vi "適應性控制_連續取樣版(實際控制).vi"() -> ()   [LabVIEW 2010]
panel:
  out "A1_input_x(t)":dbl(graph)
  in  "milliseconds to wait":u32
  out "Numeric":dbl
  out "while平均運行時間(ms)":dbl
  in  "number of samples(不可低於2)":i32=100 min=2
  in  "rate":dbl=1000.0
  out "收斂時間(s)":dbl
  out "收斂燈":bool
  in  "ERR誤差低於多少V亮燈":dbl=0.05
  out "ERR message":string=" INSTRUCTIONS:\r\rNormal Use:  When using subVIs that incorporate the error in/error out (or error I/O) structure, place this handler where you want to inform the user of an error, typically at the end of the I/O data path, as the last action of the program.  If the error in error? is ERROR, the handler creates a message describing the error and its source.  If the type of dialog = 1 (default), the message is displayed to the user, who can only acknowedge it.  If the type = 2, the user can acknowledge the message or abort execution; aborting a program with active I/O is not recommended.  If the type = 0, no message is displayed; this is used to process the error programmatically, and the error out cluster elements are wired to individual terminals for that reason.  \r\rOther Use:\n\r\nlocal testing.  To test the error code of a subVI or function that does not have the error I/O structure, you can wire its error code and a source string to the local error code and error source inputs.  If error in error? indicates no error and error code is not equal to 0, the local code and source are substituted for the error in values, and error? is set TRUE (ERROR)."
  out "理想系統與FIR輸出":cluster{dbl, dbl}(graph)
  out "system輸出":dbl
  out "A0_input_x(t)":dbl(graph)
  out "ERR":dbl(graph)
  out "權重函數向量":dbl[](array[numeric])
  in  "order":i32=8
  out "LMS":dbl[](graph)
  out "FIR輸出":dbl
  in  "Stop Button":bool
  in  "u(收斂係數)":dbl=0.005
  # "A0:模擬輸入 pulse_output 1"
  # "A1:理想系統 pulse_output 2"
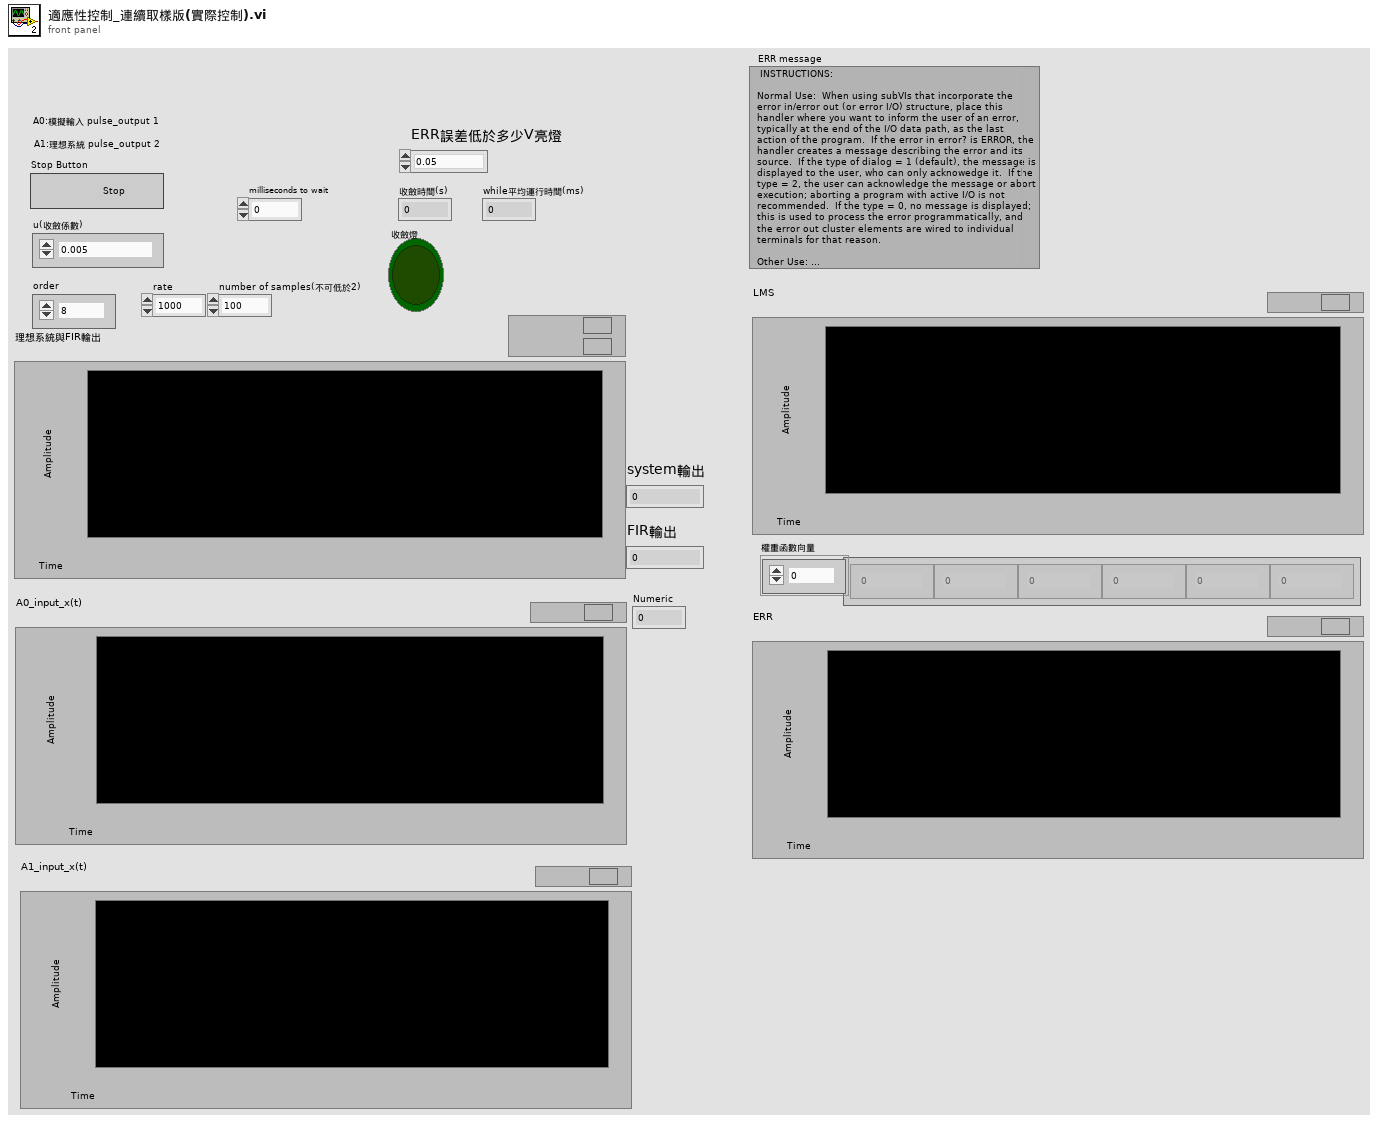
[diagram p1: front panel]
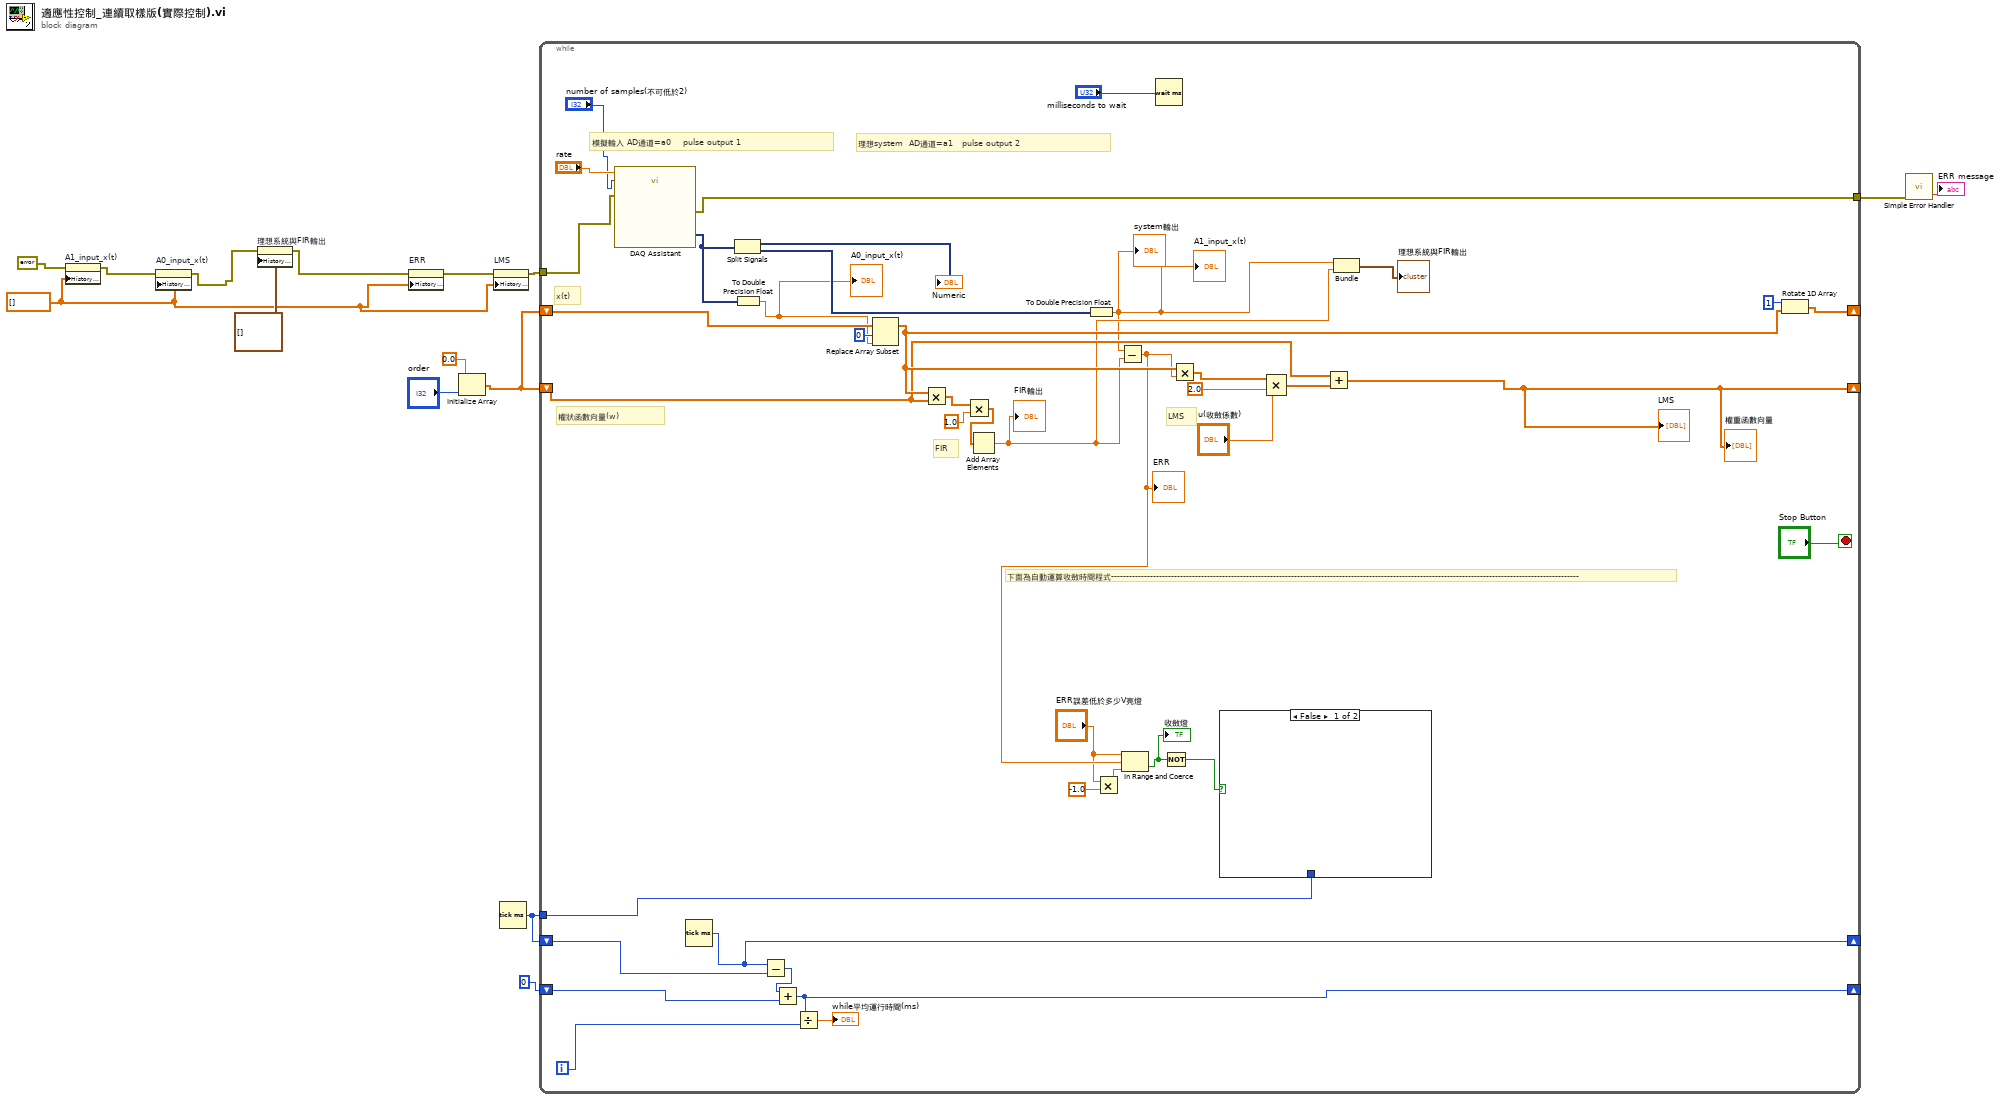
[diagram p0: block diagram]
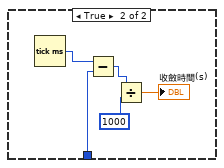
[diagram p2: hidden frame]
diagram:
  w1 = dbl[] [] ("History Data")
  n1 = property on="A1_input_x(t)" class="WFChart (strict)"(error in=errorcluster {"status"=FALSE, "code"=0, "source"=""} ("error constant"), "History Data"=w1) -> (error out=w2:errorcluster)  [unwired: 1 in, 1 out]
  n2 = property on="A0_input_x(t)" class="WFChart (strict)"(error in=w2, "History Data"=w1) -> (error out=w10:errorcluster)  [unwired: 1 in, 1 out]
  n3 = property on="理想系統與FIR輸出" class="WFChart (strict)"(error in=w10, "History Data"=cluster{dbl, dbl}[] []) -> (error out=w9:errorcluster)  [unwired: 1 in, 1 out]
  n4 = property on="ERR" class="WFChart (strict)"(error in=w9, "History Data"=w1) -> (error out=w11:errorcluster)  [unwired: 1 in, 1 out]
  n5 = Initialize Array "Initialize Array"(0.0 ("element"), "order") -> (w13:dbl[])
  n6 = property on="LMS" class="WFChart (strict)"(error in=w11, "History Data"=w1) -> (error out=w12:errorcluster)  [unwired: 1 in, 1 out]
  n7 = Tick Count (ms)() -> (millisecond timer value=w5:u32)
  n8 = while {
    shift-right: [w47] -> _
    shift-left: w13 -> [w46]
    shift-right: [w43] -> _
    shift-left: w13 -> [w42]
    tunnel: w12 -> [w41]
    tunnel: [w19] -> w7
    shift-right: [w29] -> _
    shift-left: w5 -> [w31]
    tunnel: w5 -> [w30]
    shift-right: [w23] -> _
    shift-left: u32 0 ("y") -> [w24]
    i -> [w27]
    stop <- "Stop Button" stop-if-true
    # "下面為自動運算收斂時間程式------------------------------------------------------------------------------------------------------------------------------------------------------------"
    # "LMS"
    # "FIR"
    # "模擬輸入 AD通道=a0    pulse output 1"
    # "權狀函數向量(w)"
    # "x(t)"
    # "理想system  AD通道=a1   pulse output 2"
    n9 = call "DAQ Assistant"("rate"="rate", "number of samples"="number of samples(不可低於2)", "error in"=w41) -> ("data"=w22:dynamicdata, "error out"=w19:errorcluster)  [unwired: 13 in, 2 out]
    n10 = Tick Count (ms)() -> (millisecond timer value=w29:u32)
    n11 = Split Signals(w22) -> (→"Numeric":dynamicdata, w20:dynamicdata)  [unwired: 2 in]
    n12 = To Double Precision Float(number=w22) -> (double precision float=w16:dbl)
    "A0_input_x(t)" <- w16
    n13 = Subtract(x=w29, y=w31) -> (x-y=w25:u32)
    n14 = Add(x=w25, y=w24) -> (x+y=w23:u32)
    n15 = Divide(x=w23, y=w27) -> (x/y=→"while平均運行時間(ms)":dbl)
    n16 = Replace Array Subset "Replace Array Subset"(array=w46, new element=w16, index=0) -> (w44:dbl[])
    n17 = Multiply(x=w44, y=w42) -> (x*y=w56:dbl[])
    n18 = Multiply(x=w56, y=1.0) -> (x*y=w49:dbl[])
    n19 = Add Array Elements(numeric array=w49) -> (sum=w40:dbl)
    "FIR輸出" <- w40
    n20 = To Double Precision Float(number=w20) -> (double precision float=w17:dbl)
    "system輸出" <- w17
    "A1_input_x(t)" <- w17
    n21 = Multiply(x="ERR誤差低於多少V亮燈", y=-1.0) -> (x*y=w37:dbl)
    n22 = Subtract(x=w17, y=w40) -> (x-y=w38:dbl)
    "ERR" <- w38
    n23 = In Range and Coerce(upper limit="ERR誤差低於多少V亮燈", x=w38, lower limit=w37) -> (In Range?=w33:bool)  [unwired: 1 out]
    "收斂燈" <- w33
    n24 = Wait (ms)(milliseconds to wait="milliseconds to wait") -> ()  [unwired: 1 out]
    n25 = Not(x=w33) -> (.not. x?=w34:bool)
    n26 = Multiply(x=w44, y=w38) -> (x*y=w54:dbl[])
    n27 = case shown="False" w34 {
      tunnel: w30 -> [_ w60]
      frame False {
      }
      frame True {
        n28 = Tick Count (ms)() -> (millisecond timer value=w61:u32)
        n29 = Subtract(x=w61, y=w60) -> (x-y=w59:u32)
        n30 = Divide(x=w59, y=u32 1000) -> (x/y=→"收斂時間(s)":dbl)
      }
    }
    n31 = Compound Arithmetic op=MULTIPLY(w54, 2.0 ("value"), "u(收斂係數)") -> (w51:dbl[])
    n32 = Add(x=w42, y=w51) -> (x+y=w43:dbl[])
    "LMS" <- w43
    "權重函數向量" <- w43
    n33 = Bundle(w17, w40) -> (→"理想系統與FIR輸出":cluster{dbl, dbl})  [unwired: 1 in]
    n34 = Rotate 1D Array(1:w44, 2:1 ("n")) -> (0:w47:dbl[])
  }
  n35 = call <vilib>:"Simple Error Handler.vi"("error in (no error)"=w7) -> ("message"=→"ERR message":string)  [unwired: 4 in, 4 out]
